vi "Write Item Names.vi"(8 "error in (no error)":errorcluster, 10 "Item Names":string[][](array[string]), 11 "MCLBControl in":refnum<class "MulticolumnListboxSelection.lvclass">) -> (0 "error out":errorcluster, 3 "MCLBControl out":refnum<class "MulticolumnListboxSelection.lvclass">)   [LabVIEW 2015, in "MulticolumnListboxSelection.lvclass"]
doc: "This VI is an override of the Item Names property. It defaults all items to also have the False Symbol.\n<b> </b> <b> </b>\n©2016 Q Software Innovations, LLC (QSI)\nwritten by Quentin Alldredge\nproduced in LabVIEW 2015\n\nsupport@qsoftwareinnovations.com\nwww.qsoftwareinnovations.com\n\nAll rights reserved.\n\nRedistribution and use in source and binary forms, with or without modification, are permitted provided that the following conditions are met:\n\n * Redistributions of source code must retain the above copyright notice, this list of conditions and the following disclaimer.\n * Redistributions in binary form must reproduce the above copyright notice, this list of conditions and the following disclaimer in the documentation and/or other materials provided with the distribution.\n * Neither the name of Q Software Innovations, LLC. nor the names of its contributors may be used to endorse or promote products derived from this software without specific prior written permission.\n\nTHIS SOFTWARE IS PROVIDED BY THE COPYRIGHT HOLDERS AND CONTRIBUTORS \"AS IS\" AND ANY EXPRESS OR IMPLIED WARRANTIES, INCLUDING, BUT NOT LIMITED TO, THE IMPLIED WARRANTIES OF MERCHANTABILITY AND FITNESS FOR A PARTICULAR PURPOSE ARE DISCLAIMED. IN NO EVENT SHALL THE COPYRIGHT OWNER OR CONTRIBUTORS BE LIABLE FOR ANY DIRECT, INDIRECT, INCIDENTAL, SPECIAL, EXEMPLARY, OR CONSEQUENTIAL DAMAGES (INCLUDING, BUT NOT LIMITED TO, PROCUREMENT OF SUBSTITUTE GOODS OR SERVICES; LOSS OF USE, DATA, OR PROFITS; OR BUSINESS INTERRUPTION) HOWEVER CAUSED AND ON ANY THEORY OF LIABILITY, WHETHER IN CONTRACT, STRICT LIABILITY, OR TORT (INCLUDING NEGLIGENCE OR OTHERWISE) ARISING IN ANY WAY OUT OF THE USE OF THIS SOFTWARE, EVEN IF ADVISED OF THE POSSIBILITY OF SUCH DAMAGE.\n----\n©2019 Q Software Innovations, LLC\nWritten by Quentin \"Q\" Alldredge\nCLA, LabVIEW Champion"
uses:
  MulticolumnListboxSelection.lvclass
  MulticolumnListboxSelection.lvclass/MulticolumnListboxSelection.ctl
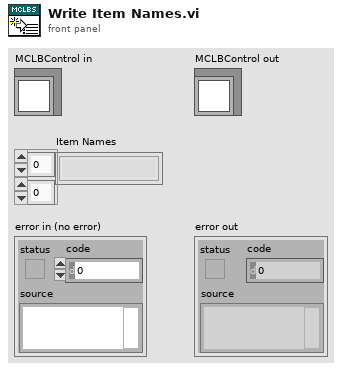
[diagram p1: front panel]
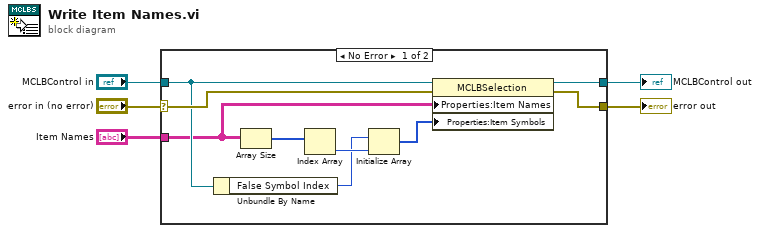
[diagram p0: block diagram]
diagram:
  n1 = case shown="No Error" "error in (no error)" {
    selector: "error in (no error)" -> [w14 w15]
    tunnel: [w6 w15] -> w5
    tunnel: [w8 w16] -> w4
    tunnel: "MCLBControl in" -> [w9 w16]
    tunnel: "Item Names" -> [w7 _]
    frame No Error {
      n2 = Unbundle By Name(w9) -> ("False Symbol Index"=w11:i32)
      n3 = Array Size(array=w7) -> (size(s)=w13:i32[])
      n4 = Index Array(array=w13) -> (element=w12:i32)  [unwired: 1 in]
      n5 = Initialize Array(w11, w12) -> (w10:i32[])
      n6 = property class="MCLBSelection"(reference=w9, error in=w14, "Properties:Item Names"=w7, "Properties:Item Symbols"=w10) -> (reference out=w8:refnum<class "MulticolumnListboxSelection.lvclass">, error out=w6:errorcluster)
    }
    frame Error {
    }
  }
  "error out" <- w5
  "MCLBControl out" <- w4
